vi "Save for Previous Version.vi"(8 "error in (no error)":errorcluster, 10 "LabVIEW Version":string, 11 "LabVIEW Library File in":refnum<class "LabVIEW Library File.lvclass">) -> (0 "error out":errorcluster, 1 "Errors":string, 2 "Warnings":string, 3 "LabVIEW Library File out":refnum<class "LabVIEW Library File.lvclass">)   [LabVIEW 2020, in "Save for Previous Version.lvlib" / "LabVIEW Library File.lvclass"]
uses:
  LabVIEW Library File.lvclass
  \\Mac\Home/JKI/GitHub/vipm-io/a-version-explorer-for-labview/experiments/save-for-previous-version/source/File/File.lvclass/File.lvclass
  File/File.lvclass/File.lvclass/File.ctl
  File/File.lvclass/Read Path.vi
  LabVIEW Library File.lvclass/LabVIEW Library File.ctl
  LabVIEW File/LabVIEW File.lvclass
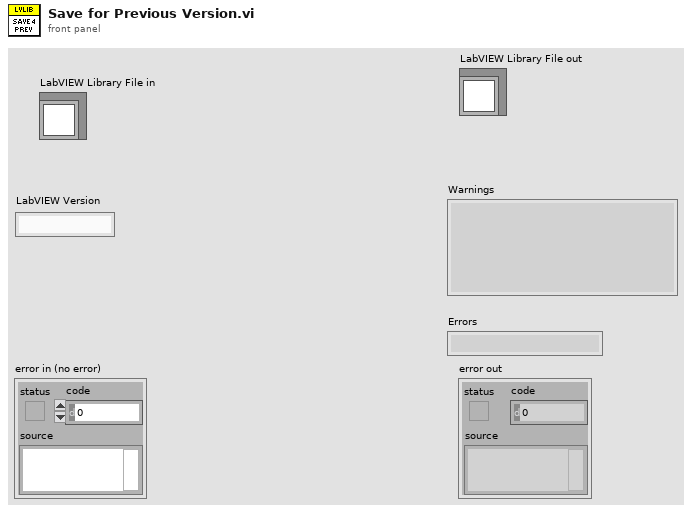
[diagram p1: front panel]
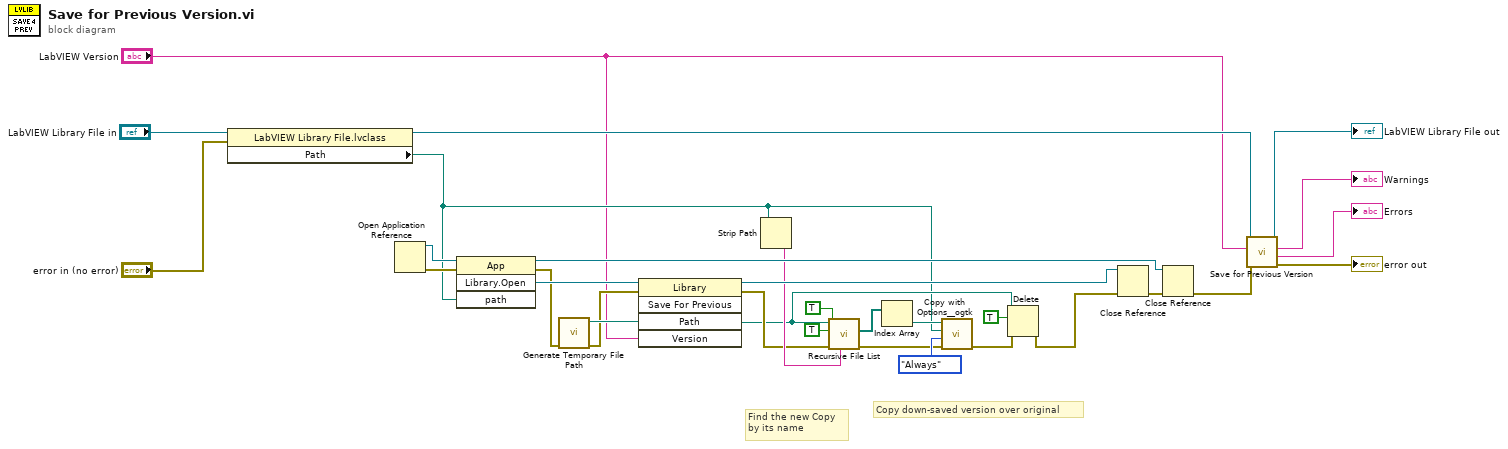
[diagram p0: block diagram]
diagram:
  # "Find the new Copy\nby its name"
  # "Copy down-saved version over original"
  n1 = property class="LabVIEW Library File.lvclass"(reference="LabVIEW Library File in", error in="error in (no error)") -> (reference out=w30:refnum<class "LabVIEW Library File.lvclass">, "Path"=w3:path)  [unwired: 1 out]
  n2 = Open Application Reference() -> (0:w23:errorcluster, 3:w22:refnum<vi>)  [unwired: 4 in]
  n3 = invoke class="App" method="Library.Open"(reference=w22, error in=w23, "path"=w3) -> (reference out=w18:refnum<vi>, error out=w5:errorcluster, "Open Library"=w21:refnum<vi>)  [unwired: 1 in, 1 out]
  n4 = call <vilib>:"Generate Temporary File Path.vi"("error in (no error)"=w5) -> ("error out"=w4:errorcluster, "Unique Temporary File Path"=w7:path)  [unwired: 9 in]
  n5 = invoke class="Library" method="Save For Previous"(reference=w21, error in=w4, "Path"=w7, "Version"="LabVIEW Version") -> (reference out=w20:refnum<vi>, error out=w10:errorcluster)  [unwired: 1 in, 3 out]
  n6 = Strip Path(path=w3) -> (name=w17:string)  [unwired: 1 out]
  n7 = call <vilib>:"Recursive File List.vi"("pattern"=w17, "error in (no error)"=w10, "Continue Recursing on Error? (F)"=TRUE, "Treat LLBs as Folders?"=TRUE, "Folder Path"=w7) -> ("error out"=w11:errorcluster, "All Files in Dir"=w14:path[])  [unwired: 2 in, 3 out]
  n8 = Index Array(array=w14) -> (element=w13:path)  [unwired: 1 in]
  n9 = call <userlib>:"Copy with Options__ogtk.vi"("error in (no error)"=w11, "Replace Mode (Never)"=enum16{"Never", "Always", "If Newer"}."Always", "target path"=w3, "source path"=w13) -> ("error out"=w9:errorcluster)  [unwired: 6 in, 1 out]
  n10 = Delete(path (use dialog)=w7, entire hierarchy (F)=TRUE, error in=w9) -> (error out=w8:errorcluster)  [unwired: 2 in, 2 out]
  n11 = Close Reference(reference=w20, error in (no error)=w8) -> (error out=w19:errorcluster)
  n12 = Close Reference(reference=w18, error in (no error)=w19) -> (error out=w1:errorcluster)
  n13 = call-parent "Save for Previous Version.vi"("error in (no error)"=w1, "LabVIEW Version"="LabVIEW Version", "LabVIEW File in"=w30) -> ("error out"=→"error out":errorcluster, "Errors"=→"Errors":string, "Warnings"=→"Warnings":string, "LabVIEW File out"=→"LabVIEW Library File out":refnum<class "LabVIEW Library File.lvclass">)  [unwired: 5 in]
